vi "Stop_Function.vi"(9 "Encoder Counts":dbl, 10 "Current Rotary Speed":dbl, 11 "Current Rotary Speed prev":dbl) -> (3 "Stop":bool)   [LabVIEW 2018]
doc: "This VI responsible for stopping the program when the rotary speed is equal to 0 for 2 readings. If 2 consecutive readings are equal to 0 and the encoder count isn't equal to zero, then the boolean \"Stop\" value is set to TRUE.\n\nInputs:\nCurrent Rotary Speed;\nCurrent Rotary Speed prev.\n\nOutputs:\n\"Stop\" boolean."
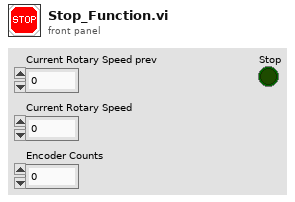
[diagram p1: front panel]
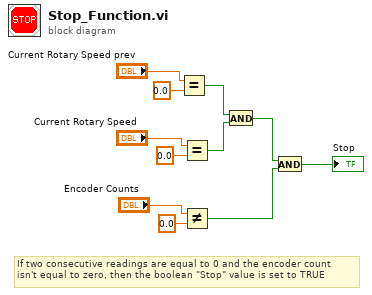
[diagram p0: block diagram]
diagram:
  # "If two consecutive readings are equal to 0 and the encoder count\nisn't equal to zero, then the boolean \"Stop\" value is set to TRUE"
  n1 = Equal?(x="Current Rotary Speed prev", y=0.0) -> (x = y?=w4:bool)
  n2 = Equal?(x="Current Rotary Speed", y=0.0) -> (x = y?=w3:bool)
  n3 = Not Equal?(x="Encoder Counts", y=0.0) -> (x != y?=w2:bool)
  n4 = And(x=w4, y=w3) -> (x .and. y?=w1:bool)
  n5 = And(x=w1, y=w2) -> (x .and. y?=→"Stop":bool)
